vi "to string 1.0.vi"(8 "error in (no error)":errorcluster, 10 "data in":string, 11 "UI Reference configuration in":refnum<class "UI Reference configuration.lvclass">) -> (0 "error out":errorcluster, 2 "data out":string, 3 "UI Reference configuration out":refnum<class "UI Reference configuration.lvclass">)   [LabVIEW 2014, in "UI Reference configuration.lvclass"]
uses:
  UI Reference configuration.lvclass
  UI Reference configuration.lvclass/UI Reference configuration.ctl
  <vilib>/NI/Tag Bus Module Framework/channel/TBM channel.lvclass
  <vilib>/NI/Configuration Framework/serializable configuration/NISE_CEF_serializable configuration.lvclass
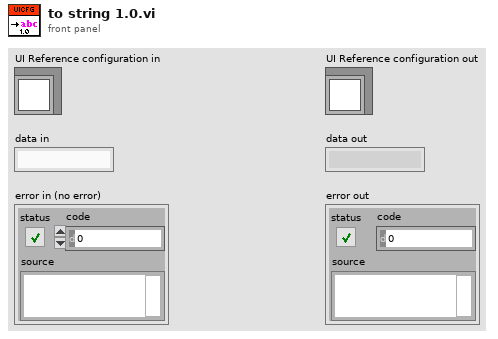
[diagram p1: front panel]
types:
  T1 = typedef "UI Reference configuration.lvclass/Line.ctl" = cluster{"channel":refnum<class "TBM channel.lvclass">}
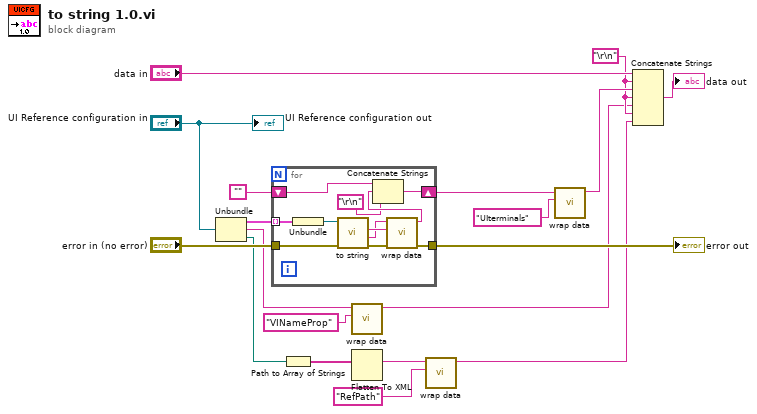
[diagram p0: block diagram]
diagram:
  w3 = "\r\n"
  n1 = Unbundle("UI Reference configuration in") -> (w15:T1[], w6:string, w5:path)
  n2 = for {
    tunnel: w15 -> [w29] mode=indexing
    tunnel: "error in (no error)" -> [w25]
    tunnel: [w24] -> w19
    shift-right: [w21] -> w12
    shift-left: "" -> [w22]
    n3 = Unbundle(w29) -> ("channel"=w28:refnum<class "TBM channel.lvclass">)
    n4 = call-dynamic "to string.vi"("error in"=w25, "channel in"=w28) -> ("error out"=w24:errorcluster, "channel data"=w26:string, "identifier"=w27:string)  [unwired: 6 in, 1 out]
    n5 = call <vilib>:"wrap data.vi"("identifier"=w27, "data to wrap"=w26) -> ("wrapped data"=w23:string)  [unwired: 9 in]
    n6 = Concatenate Strings(w22, w23, "\r\n") -> (w21:string)
  }
  "error out" <- w19
  n7 = Path to Array of Strings(0:w5) -> (2:w8:string[])  [unwired: 1 out]
  n8 = call <vilib>:"wrap data.vi"("identifier"="VINameProp" ("additional identifier"), "data to wrap"=w6) -> ("wrapped data"=w2:string)  [unwired: 9 in]
  n9 = Flatten To XML(anything=w8) -> (xml string=w7:string)
  n10 = call <vilib>:"wrap data.vi"("identifier"="RefPath" ("additional identifier"), "data to wrap"=w7) -> ("wrapped data"=w1:string)  [unwired: 9 in]
  n11 = call <vilib>:"wrap data.vi"("identifier"="UIterminals" ("additional identifier"), "data to wrap"=w12) -> ("wrapped data"=w4:string)  [unwired: 9 in]
  n12 = Concatenate Strings("data in", w3, w4, w3, w2, w3, w1) -> (→"data out":string)
  "UI Reference configuration out" <- "UI Reference configuration in"
